vi "Left Aligned nodes.vi"() -> ()   [LabVIEW 2025]
uses:
  <vilib>/JDP Science/JSONtext/JSONtext.lvlib
panel:
  out "Last Event":T1
  out "Log":string[](array[string]) caption="Log (newest first)"
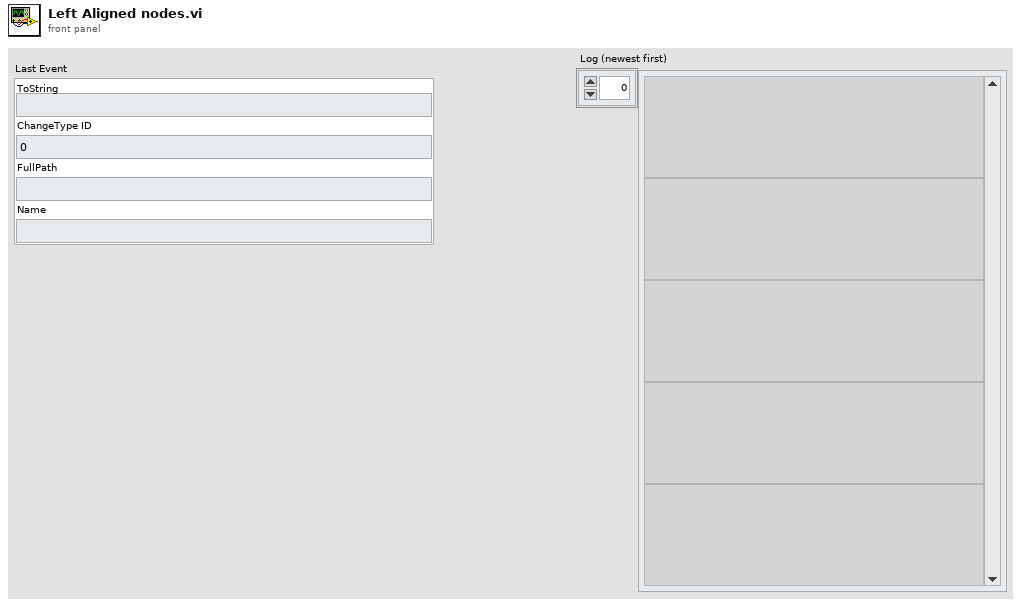
[diagram p1: front panel]
types:
  T1 = cluster{"ToString":string, "ChangeType ID":dbl, "FullPath":string, "Name":string}
  T2 = cluster{"queue out":refnum<queue>, "notifier out":refnum<notifier>}
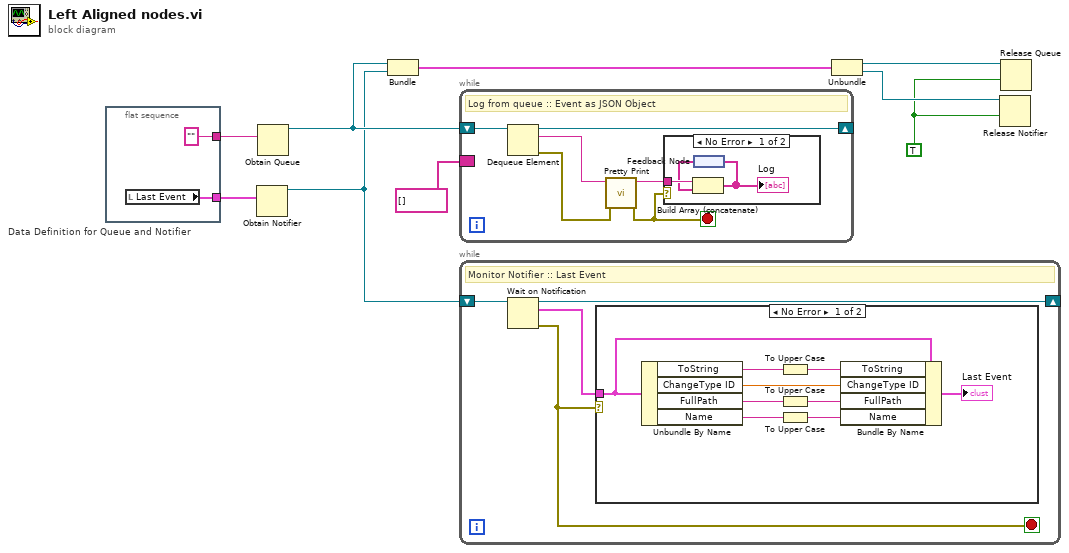
[diagram p0: block diagram]
diagram:
  w1 = TRUE ("force destroy? (F)")
  n1 = flat-sequence "Data Definition for Queue and Notifier" {
    tunnel: [w11] -> w6
    tunnel: ["" ("name (unnamed)")] -> w5
    frame #0 {
      n2 = local read "Last Event"() -> (w11:T1)
    }
  }
  n3 = Obtain Notifier(notification data type=w6) -> (notifier out=w7:refnum<notifier>)  [unwired: 3 in, 2 out]
  n4 = Obtain Queue(element data type=w5) -> (queue out=w8:refnum<queue>)  [unwired: 4 in, 2 out]
  n5 = Bundle("queue out"=w8, "notifier out"=w7) -> (w9:T2)  [unwired: 1 in]
  n6 = while {
    shift-right: [w16] -> _
    shift-left: w8 -> [w17]
    border: string[] [] -> [_]
    stop <- w13 stop-if-true
    # "Log from queue :: Event as JSON Object"
    n7 = Dequeue Element(queue=w17) -> (queue out=w16:refnum<queue>, element=w15:string, error out=w14:errorcluster)  [unwired: 2 in, 1 out]
    n8 = call <vilib>:"Pretty Print.vi"("error in (no error)"=w14, "JSON"=w15) -> ("error out"=w13:errorcluster, "<JSON>"=w12:string)  [unwired: 7 in, 1 out]
    n9 = case shown="No Error" w13 {
      tunnel: w12 -> [w20 _]
      frame No Error {
        n10 = feedback #1() -> (w18:string[])
        n11 = Build Array (concatenate)(w20, w18) -> (w19:string[])
        "Log" <- w19
        n12 = feedback-in #1(w19) -> ()
      }
      frame Error {
      }
    }
  }
  n13 = while {
    shift-right: [w23] -> _
    shift-left: w7 -> [w24]
    stop <- w21 stop-if-true
    # "Monitor Notifier :: Last Event"
    n14 = Wait on Notification(notifier=w24) -> (notifier out=w23:refnum<notifier>, notification=w22:T1, error out=w21:errorcluster)  [unwired: 3 in, 1 out]
    n15 = case shown="No Error" w21 {
      tunnel: w22 -> [w25 _]
      frame No Error {
        n16 = Unbundle By Name(w25) -> ("ToString"=w33:string, "ChangeType ID"=w30:dbl, "FullPath"=w32:string, "Name"=w31:string)
        n17 = To Upper Case(1:w33) -> (0:w27:string)
        n18 = To Upper Case(1:w32) -> (0:w29:string)
        n19 = To Upper Case(1:w31) -> (0:w28:string)
        n20 = Bundle By Name(cluster=w25, "ToString"=w27, "ChangeType ID"=w30, "FullPath"=w29, "Name"=w28) -> (→"Last Event":T1)
      }
      frame Error {
      }
    }
  }
  n21 = Unbundle(w9) -> ("queue out"=w3:refnum<queue>, "notifier out"=w2:refnum<notifier>)
  n22 = Release Notifier(notifier=w2, force destroy? (F)=w1) -> ()  [unwired: 1 in, 3 out]
  n23 = Release Queue(queue=w3, force destroy? (F)=w1) -> ()  [unwired: 1 in, 3 out]
